vi "Trace.vi"   [LabVIEW 2020, in "NI_AALPro.lvlib"]
doc: "Finds the <B>trace</B> of <B>Input Matrix</B>. Wire data to the <B>Input Matrix</B> input to determine the polymorphic instance to use or manually select the instance."
uses:
  NI_AALPro.lvlib
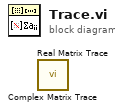
[diagram p0: block diagram]
diagram:
  n1 = call "Complex Matrix Trace.vi"() -> ()  [unwired: 1 in, 2 out]
  n2 = call "Real Matrix Trace.vi"() -> ()  [unwired: 1 in, 2 out]
